vi "measPwrCur.vi"(0 "VISA resource name":refnum<visa-resource-name>="6812B", 3 "error in (no error)":errorcluster) -> (1 "PwrMeas":T1, 4 "CurMeas":T2, 5 "VISA resource name out":refnum<visa-resource-name>, 8 "error out":errorcluster)   [LabVIEW 2019]
uses:
  <instrlib>/Agilent 681x Series/Public/Data/Read Single Measurement (Current).vi
  <instrlib>/Agilent 681x Series/Public/Data/Low Level/Fetch Single Measurement (Power).vi
  <instrlib>/Agilent 681x Series/Agilent 681x Series.lvlib
panel:
  in  "Relative Trigger Samples (0)":i32
  in  "Sample Spacing (25 us)":dbl=2.5e-05 format="%^.2g"
  in  "Maximum Time (10000 ms)":i32=10000
  in  "Sense Source (0: Internal)":u16(ring) items=["Internal", "External"]
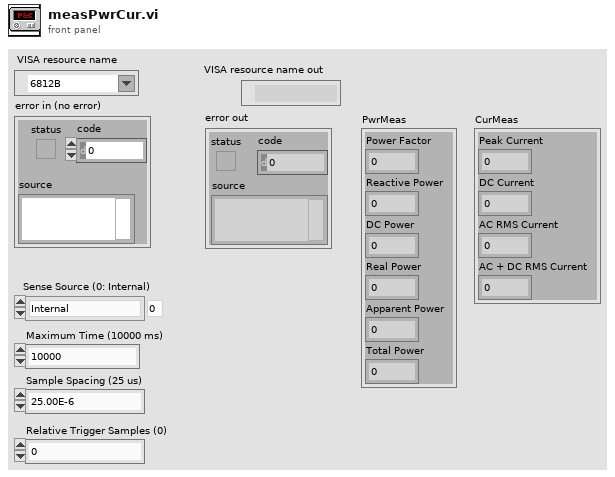
[diagram p1: front panel]
types:
  T1 = cluster{"Power Factor":dbl, "Reactive Power":dbl, "DC Power":dbl, "Real Power":dbl, "Apparent Power":dbl, "Total Power":dbl}
  T2 = cluster{"Peak Current":dbl, "DC Current":dbl, "AC RMS Current":dbl, "AC + DC RMS Current":dbl}
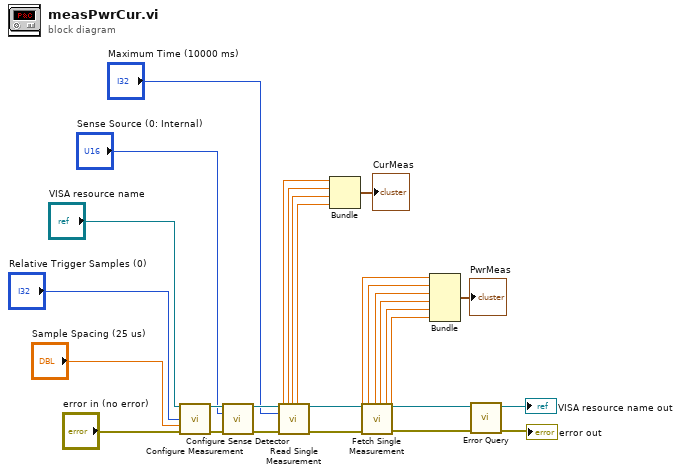
[diagram p0: block diagram]
diagram:
  n1 = call <instrlib>:"Configure Measurement.vi"("VISA resource name"="VISA resource name", "Relative Trigger Samples (0)"="Relative Trigger Samples (0)", "Sample Spacing (25 us)"="Sample Spacing (25 us)", "error in (no error)"="error in (no error)") -> ("VISA resource name out"=w24:refnum<visa-resource-name>, "error out"=w23:errorcluster)  [unwired: 10 in]
  n2 = call <instrlib>:"Configure Sense Detector.vi"("VISA resource name"=w24, "Sense Source (0: Internal)"="Sense Source (0: Internal)", "error in (no error)"=w23) -> ("VISA resource name out"=w26:refnum<visa-resource-name>, "error out"=w25:errorcluster)  [unwired: 11 in]
  n3 = call-poly <instrlib>:"Read Single Measurement.vi"("VISA resource name"=w26, "Maximum Time (10000 ms)"="Maximum Time (10000 ms)", "error in (no error)"=w25) -> ("Peak Current"=w12:dbl, "VISA resource name out"=w27:refnum<visa-resource-name>, "DC Current"=w11:dbl, "AC RMS Current"=w10:dbl, "AC + DC RMS Current"=w9:dbl, "error out"=w28:errorcluster)  [unwired: 7 in]
  n4 = Bundle("Peak Current"=w12, "DC Current"=w11, "AC RMS Current"=w10, "AC + DC RMS Current"=w9) -> (→"CurMeas":T2)  [unwired: 1 in]
  n5 = call-poly <instrlib>:"Fetch Single Measurement.vi"("VISA resource name"=w27, "error in (no error)"=w28) -> ("Power Factor"=w7:dbl, "Reactive Power"=w6:dbl, "VISA resource name out"=w16:refnum<visa-resource-name>, "DC Power"=w5:dbl, "Real Power"=w4:dbl, "Apparent Power"=w3:dbl, "Total Power"=w2:dbl, "error out"=w15:errorcluster)  [unwired: 6 in]
  n6 = Bundle("Power Factor"=w7, "Reactive Power"=w6, "DC Power"=w5, "Real Power"=w4, "Apparent Power"=w3, "Total Power"=w2) -> (→"PwrMeas":T1)  [unwired: 1 in]
  n7 = call <instrlib>:"Error Query.vi"("error in (no error)"=w15, "VISA resource name"=w16) -> ("error out"=→"error out":errorcluster, "VISA resource name out"=→"VISA resource name out":refnum<visa-resource-name>)  [unwired: 6 in, 2 out]
